vi "ReadSV.vi"(8 "error in (no error)":errorcluster, 11 "shared variable refnum":refnum<k21>) -> (0 "error out":errorcluster, 2 "DBL Data":dbl)   [LabVIEW 2020, in "Shared Variable Interface.lvlib" / "DBL.lvlib"]
uses:
  DBL.lvlib
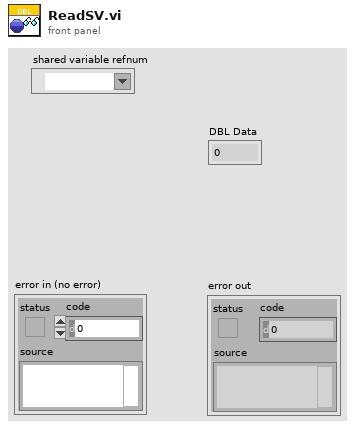
[diagram p1: front panel]
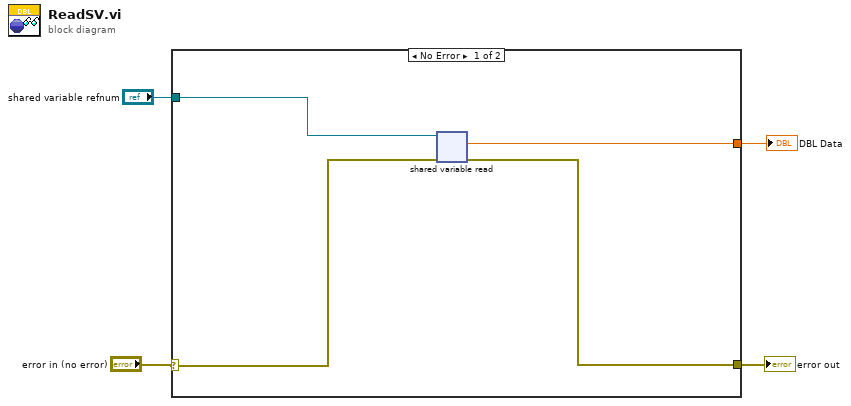
[diagram p0: block diagram]
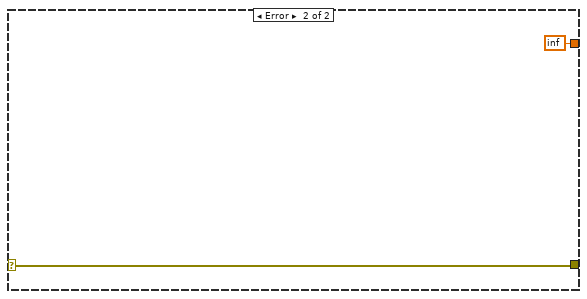
[diagram p2: hidden frame]
diagram:
  n1 = case shown="No Error" "error in (no error)" {
    selector: "error in (no error)" -> [w6 w10]
    tunnel: [w8 w10] -> w4
    tunnel: [w7 inf] -> w2
    tunnel: "shared variable refnum" -> [w5 _]
    frame No Error {
      n2 = shared-variable-read(w5, w6) -> (w8:errorcluster, w7:dbl)  [unwired: 2 out]
    }
    frame Error {
    }
  }
  "error out" <- w4
  "DBL Data" <- w2
